vi "Read Pin.vi"(6 "Pin":u16, 8 "error in (no error)":errorcluster, 9 "Port":u16, 10 "VISA resource name":refnum<visa-resource-name>, 11 "Simulada in":refnum<class "Simulada.lvclass">) -> (0 "error out":errorcluster, 1 "Boolean":bool, 2 "VISA resource name 2":refnum<visa-resource-name>, 3 "Simulada out":refnum<class "Simulada.lvclass">)   [LabVIEW 2020, in "Simulada.lvclass"]
uses:
  Simulada.lvclass
  Abstract/Serial Device/Serial Device.lvclass
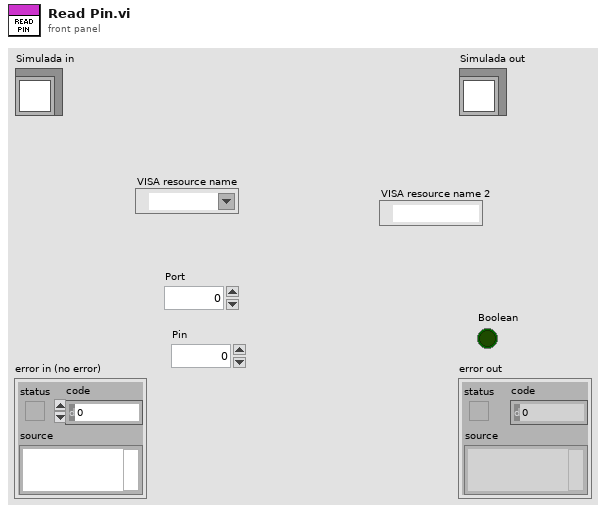
[diagram p1: front panel]
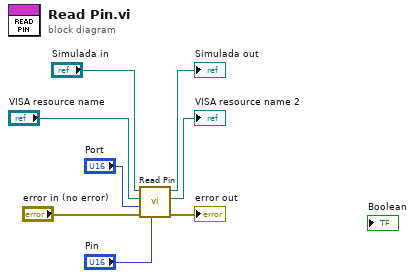
[diagram p0: block diagram]
diagram:
  n1 = call-parent "Read Pin.vi"("Pin"="Pin", "error in (no error)"="error in (no error)", "Port"="Port", "VISA resource name"="VISA resource name", "Serial Device in"="Simulada in") -> ("error out"=→"error out":errorcluster, "VISA resource name 2"=→"VISA resource name 2":refnum<visa-resource-name>, "Serial Device out"=→"Simulada out":refnum<class "Simulada.lvclass">)  [unwired: 3 in, 1 out]
